vi "Close.vi"(8 "error in (no error)":errorcluster) -> (0 "error out":errorcluster)   [LabVIEW 2019, in "maxonEPOS.lvlib"]
doc: "<B>Close</B> closes all opened ports and releases it for other applications."
uses:
  Examples/maxonEPOS.lvlib
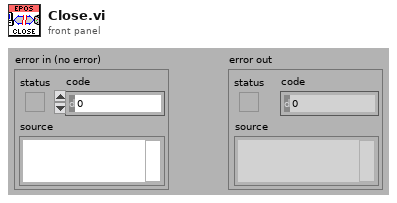
[diagram p1: front panel]
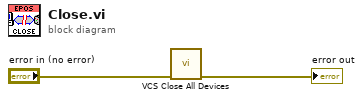
[diagram p0: block diagram]
diagram:
  n1 = call "VCS Close All Devices.vi"("error in (no error)"="error in (no error)") -> ("error out"=→"error out":errorcluster)  [unwired: 10 in]
